vi "main.vi"() -> ()   [LabVIEW 2019]
uses:
  <vilib>/myRIO/Instrument Drivers/Onboard IO/I2C/typedefs/I2C Transfer Rate.ctl
  <vilib>/myRIO/Instrument Drivers/Onboard IO/I2C/I2C.lvlib
  <vilib>/myRIO/Instrument Drivers/Onboard IO/I2C/typedefs/I2C User Configuration.ctl
  <vilib>/myRIO/Instrument Drivers/Onboard IO/I2C/typedefs/I2C Configuration.ctl
  <vilib>/myRIO/Common/Instrument Driver Framework/myRIO v1.0/I2C/typedefs/I2C Channels Enum.ctl
  <vilib>/myRIO/Common/Instrument Driver Framework/Utilities/typedefs/Generic FPGA Reference.ctl
  <vilib>/myRIO/Common/Instrument Driver Framework/Utilities/typedefs/myRIO v1.0 Reference.ctl
  <vilib>/myRIO/Common/Instrument Driver Framework/Utilities/typedefs/Hardware Version Enum.ctl
  <vilib>/myRIO/Common/Instrument Driver Framework/Utilities/typedefs/myRIO Generic Hardware Reference.ctl
  <vilib>/myRIO/Instrument Drivers/Onboard IO/I2C/typedefs/I2C Reference.ctl
  <vilib>/myRIO/Instrument Drivers/Onboard IO/I2C/vis/Configure.vi
  <vilib>/userDefined/High Color/nirio_resource_hc.ctl
  <vilib>/myRIO/Common/Instrument Driver Framework/myRIO v1.0/I2C/vis/myRIO v1.1 Open I2C.vi
  <vilib>/myRIO/Instrument Drivers/Onboard IO/I2C/vis/myRIO I2C Open.xnode
  <vilib>/myRIO/Common/Instrument Driver Framework/Utilities/vis/Is FPGA Ref Available.vi
  <vilib>/myRIO/Express VI/Onboard IO/I2C/I2C Express VI.xnode
  <vilib>/Platform/TimedLoop/XDataNode/wakeup.ctl
  <vilib>/Platform/TimedLoop/XDataNode/XDNodeRunTimeDep.lvlib
  <vilib>/Platform/TimedLoop/XDataNode/nitl_modes.ctl
  <vilib>/Platform/TimedLoop/XDataNode/timing_clust.ctl
  <vilib>/platform/TimedLoop/XDataNode/XDataNode.xnode
  <vilib>/myRIO/Instrument Drivers/Onboard IO/I2C/vis/Write Read.vi
  <vilib>/myRIO/Instrument Drivers/Onboard IO/I2C/vis/Write.vi
  <vilib>/myRIO/Instrument Drivers/Utilities/Utilities.lvlib
  <vilib>/myRIO/Instrument Drivers/Onboard IO/PWM/PWM.lvlib
  <vilib>/myRIO/Instrument Drivers/Onboard IO/PWM/vis/myRIO PWM Open.xnode
  <vilib>/myRIO/Instrument Drivers/Onboard IO/PWM/typedefs/PWM Reference.ctl
  <vilib>/myRIO/Instrument Drivers/Onboard IO/PWM/typedefs/PWM Configuration.ctl
  <vilib>/myRIO/Common/Instrument Driver Framework/myRIO v1.0/PWM/typedefs/PWM Channels Enum.ctl
  <vilib>/myRIO/Common/Instrument Driver Framework/myRIO v1.0/PWM/vis/myRIO v1.1 Open PWM.vi
  OneDrive/Documents/LabVIEW Data/MathScriptVIs/MCStatic_41946317732_98df4686c37d1a1eae0c5985e9f7cbe2.vi
  <vilib>/imath/engines/lvmath2/RunTimeEngine/ArithmeticOperatorToken/NIMS_ArithmeticOperator_multmx.vi
  <vilib>/imathl/engines/lvmath/Functions/Error Handling/Create Error.vi
  <vilib>/imath/engines/lvmath/Functions/Error Handling/MergeErrorsWrapper.vi
  <vilib>/imath/engines/lvmath2/RunTimeEngine/CommandStatement/MC_CommandStatement_break.vi
  OneDrive/Documents/LabVIEW Data/MathScriptVIs/MCStatic_41946317732_460fc674ac509ba7029ac98c4ab25738.vi
  <vilib>/imath/engines/lvmath2/RunTimeEngine/ArithmeticOperatorToken/NIMS_ArithmeticOperator_minus.vi
  <vilib>/imath/engines/lvmath2/RunTimeEngine/ErrorHandling/NIMS_Create Error From Enums.vi
  <vilib>/imath/engines/lvmath2/RunTimeEngine/BuiltInFunctions/abs/NIMS_abs(signed).vi
  <vilib>/imath/engines/lvmath2/RunTimeEngine/BuiltInFunctions/max/1 input/NIMS_max(RM).vi
  <vilib>/imath/engines/lvmath2/RunTimeSupport/NIMS_Get Scalar_w Error.vi
  <vilib>/imath/engines/lvmath2/RunTimeEngine/BuiltInFunctions/eye/NIMS_M=eye(I32).vi
  <vilib>/imath/engines/lvmath2/RunTimeEngine/ArithmeticOperatorToken/NIMS_ArithmeticOperator_plus.vi
  <vilib>/imath/engines/lvmath2/RunTimeEngine/BuiltInFunctions/all/NIMS_all(GM).vi
  <vilib>/imath/engines/lvmath2/RunTimeEngine/ArithmeticOperatorToken/NIMS_ArithmeticOperator_powermx(M,M).vi
  <vilib>/imath/engines/lvmath2/RunTimeEngine/CommandStatement/NIMS_CommandStatement_MaskErr.vi
  <vilib>/imath/engines/lvmath2/RunTimeEngine/ErrorHandling/NIMS_Finalize Error.vi
  Analytic_Jacobian_Mag_cir_array_test.m
  PM_forward_field.m
  <vilib>/Utility/file.llb/Write Delimited Spreadsheet (DBL).vi
  <vilib>/imath/engines/lvmath2/RunTimeEngine/BuiltInFunctions/max/1 input/NIMS_max(CM).vi
  <vilib>/imath/engines/lvmath2/RunTimeEngine/BuiltInFunctions/diag/NIMS_diag.vi
  <vilib>/imath/engines/lvmath2/RunTimeEngine/BuiltInFunctions/is_finite/NIMS_is_finite.vi
  <vilib>/imath/engines/lvmath2/RunTimeEngine/BuiltInFunctions/length/NIMS_length(GV).vi
  <vilib>/imath/engines/lvmath2/RunTimeEngine/BuiltInFunctions/norm/NIMS_norm(GM,DBL).vi
  <vilib>/imath/engines/lvmath2/RunTimeEngine/ArithmeticOperatorToken/NIMS_ArithmeticOperator_rightdivmx(C,C).vi
  <vilib>/imath/engines/lvmath2/RunTimeEngine/BuiltInFunctions/max/2 inputs/NIMS_max(CG,CG)-no size check.vi
  <vilib>/imath/engines/lvmath2/RunTimeEngine/NodeEndStatement/NIMS_NodeEndStatement_Output.vi
  <vilib>/imath/engines/lvmath2/RunTimeEngine/ArithmeticOperatorToken/NIMS_ArithmeticOperator_rightdiv.vi
  <vilib>/imath/engines/lvmath2/RunTimeEngine/ArithmeticOperatorToken/NIMS_ArithmeticOperator_leftdivmx(C,C).vi
  <vilib>/imath/engines/lvmath2/RunTimeEngine/BuiltInFunctions/mirrorh/NIMS_mirrorh(GM).vi
  <vilib>/imath/engines/lvmath2/RunTimeEngine/RowToken/NIMS_RowToken_M_M.vi
  <vilib>/Utility/file.llb/Write Delimited Spreadsheet (string).vi
  <vilib>/myRIO/Express VI/Onboard IO/PWM/PWM Express VI.xnode
  <vilib>/myRIO/Instrument Drivers/Onboard IO/PWM/vis/Set Duty Cycle and Frequency.vi
panel:
  out "pm_hat_opt 2":dbl[][](array[numeric])
  in  "stop 2":bool
  out "Combined Output":cluster{dbl, dbl, dbl, dbl, dbl, dbl}(graph) caption="Waveform Chart"
  out "MUX 2":cluster{dbl, dbl, dbl}(graph) caption="Waveform Chart"
  out "MUX 1":cluster{dbl, dbl, dbl}(graph) caption="Waveform Chart"
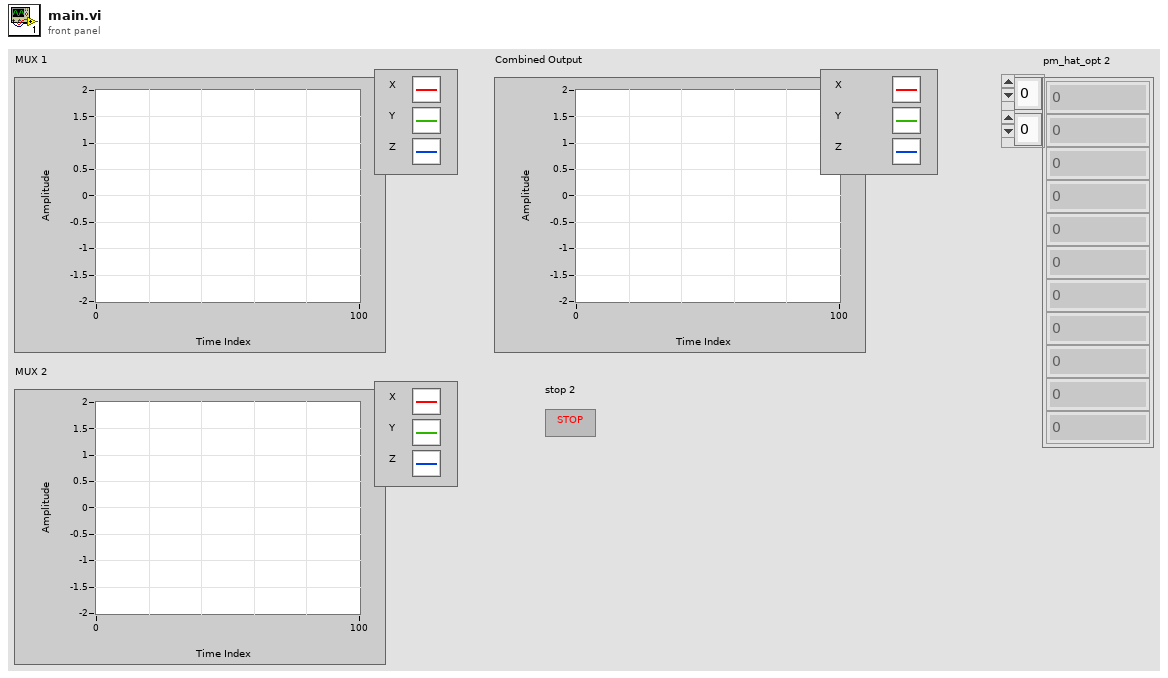
[diagram p1: front panel]
types:
  T1 = typedef "I2C.lvlib/I2C Reference.ctl" = cluster{"myRIO Reference":T2, "I2C Channels Enum":T6, "I2C Configuration":T7}
  T2 = typedef "myRIO Generic Hardware Reference.ctl" = cluster{"myRIO Model":T3, "myRIO Hardware Reference":T4}
  T3 = typedef "Hardware Version Enum.ctl" = enum16{"Unknown", "myRIO-1900", "myRIO-1950", "roboRIO", "NI ELVIS RIO CM", "ELVIS III"}
  T4 = typedef "myRIO v1.0 Reference.ctl" = cluster{"Generic FPGA Reference":T5, "Allow multiple opens":bool}
  T5 = typedef "Generic FPGA Reference.ctl" = refnum<k20>
  T6 = typedef "I2C Channels Enum.ctl" = enum16{"Not Connected", "A/I2C", "B/I2C", "I2C/I2C"}
  T7 = typedef "I2C.lvlib/I2C Configuration.ctl" = cluster{"I2C Transfer Rate":T8}
  T8 = typedef "I2C.lvlib/I2C Transfer Rate.ctl" = enum16{"Standard mode (100 kbps)", "Fast mode (400 kbps)"}
  T9 = typedef "I2C.lvlib/I2C User Configuration.ctl" = cluster{"I2C Transfer Rate":T8}
  T10 = typedef "nirio_resource_hc.ctl" = tag
  T11 = typedef "PWM.lvlib/PWM Reference.ctl" = cluster{"myRIO Reference":T2, "PWM Channels Enum":T12, "PWM Configuration":T13}
  T12 = typedef "PWM Channels Enum.ctl" = enum16{"Not Connected", "C/PWM0", "C/PWM1", "A/PWM0", "A/PWM1", "A/PWM2", "A/PWM3", "A/PWM4", "A/PWM5", "A/PWM6", "A/PWM7", "A/PWM8", "A/PWM9", "A/PWM10", "A/PWM11", "A/PWM12", "A/PWM13", "A/PWM14", "A/PWM15", "A/PWM16", "A/PWM17", "A/PWM18", "A/PWM19", "B/PWM0", "B/PWM1", "B/PWM2", "B/PWM3", "B/PWM4", "B/PWM5", "B/PWM6", "B/PWM7", "B/PWM8", "B/PWM9", "B/PWM10", "B/PWM11", "B/PWM12", "B/PWM13", "B/PWM14", "B/PWM15", "B/PWM16", "B/PWM17", "B/PWM18", "B/PWM19", "PWM/PWM0", "PWM/PWM1", "PWM/PWM2", "PWM/PWM3", "PWM/PWM4", "PWM/PWM5", "PWM/PWM6", "PWM/PWM7", "PWM/PWM8", "PWM/PWM9"}
  T13 = typedef "PWM.lvlib/PWM Configuration.ctl" = cluster{"Frequency":dbl, "Duty Cycle":dbl}
  T14 = typedef "XDNodeRunTimeDep.lvlib/timing_clust.ctl" = cluster{"Expected End [f-1]":u64, "Actual End [f-1]":u64, "Finished Late? [f-1]":bool, "Expected End [i-1]":u64, "Actual End [i-1]":u64, "Finished Late? [i-1]":bool, "Expected Start [i]":u64, "Actual Start [i]":u64, "Expected Start [f]":u64, "Actual Start [f]":u64, "Source Name":string, "Structure Name":string, "Period":i64, "Deadline":i64, "Offset":i64, "Start":i64, "Priority":i32, "Timeout":i32, "Mode":T15, "Wakeup Reason":T16, "Error":errorcluster, "Source Type":string, "Secondary Source Type":string, "Global End Time":u64, "Global Start Time":u64, "Frame Duration":u64, "Iteration Duration":u64, "Assigned CPU":i32, "I/O Scan Engine Mode":u32}
  T15 = typedef "XDNodeRunTimeDep.lvlib/nitl_modes.ctl" = enum32{"No Change", "Process missed periods, maintain original phase", "Discard missed periods, maintain original phase", "Process missed periods, ignore original phase", "Discard missed periods, ignore original phase"}
  T16 = typedef "XDNodeRunTimeDep.lvlib/wakeup.ctl" = enum32{"Normal", "Aborted", "Asynchronous wakeup", "Timing source error", "Timed loop error", "Timeout"}
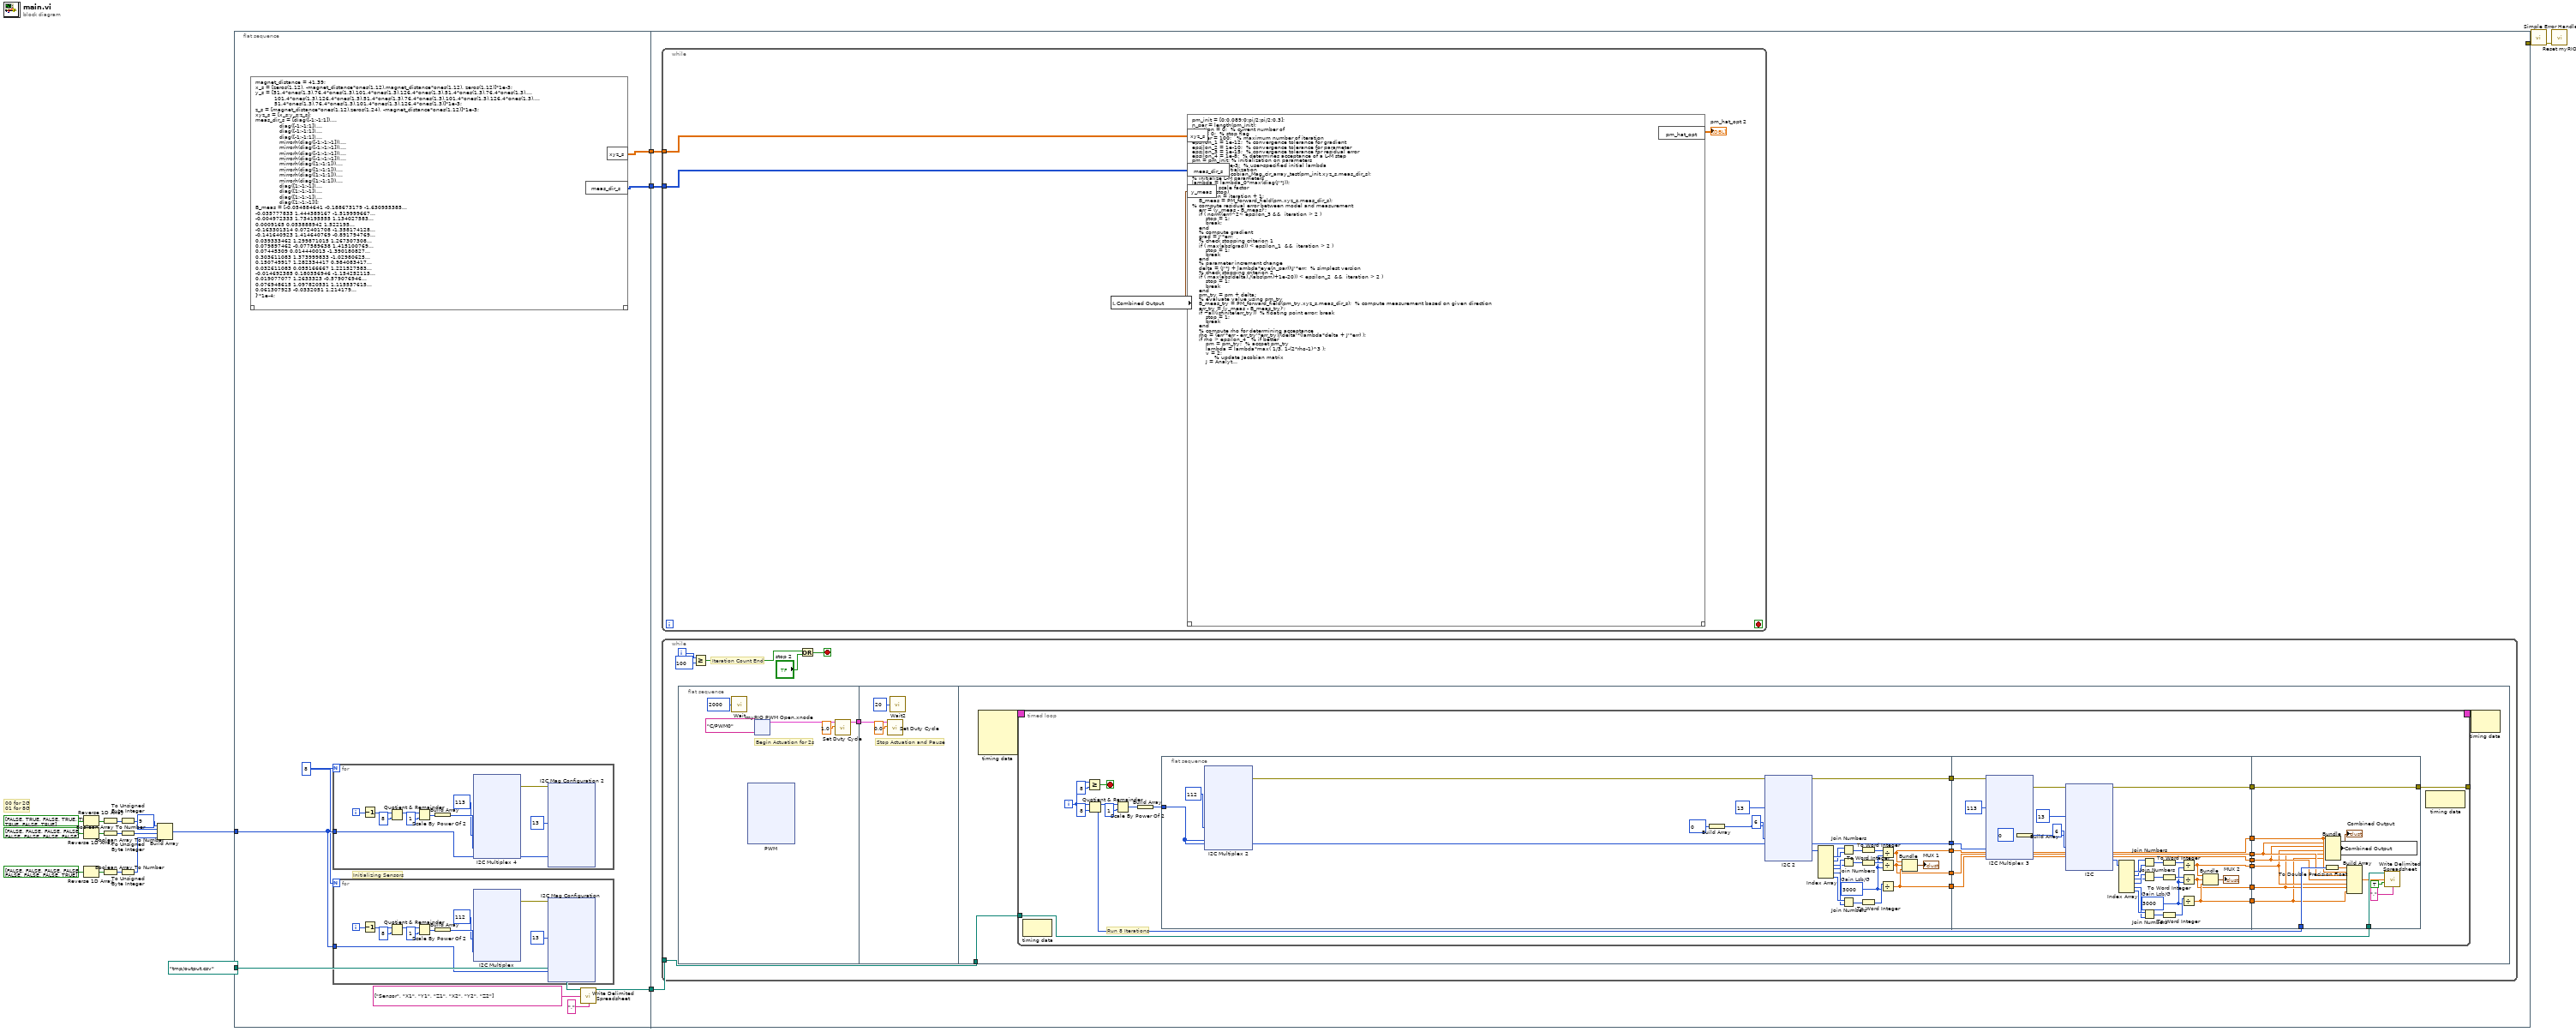
[diagram p0: block diagram]
diagram:
  # "00 for 2G\n01 for 8G"
  n1 = Reverse 1D Array(array=bool[] [FALSE, TRUE, FALSE, TRUE, TRUE, TRUE, FALSE, TRUE]) -> (reversed array=w19:bool[])
  n2 = Reverse 1D Array(array=bool[] [FALSE, FALSE, FALSE, FALSE, FALSE, FALSE, FALSE, FALSE]) -> (reversed array=w18:bool[])
  n3 = Reverse 1D Array(array=bool[] [FALSE, FALSE, FALSE, FALSE, FALSE, FALSE, FALSE, TRUE]) -> (reversed array=w16:bool[])
  n4 = Boolean Array To Number(Boolean array=w19) -> (number=w13:u32)
  n5 = Boolean Array To Number(Boolean array=w18) -> (number=w12:u32)
  n6 = Boolean Array To Number(Boolean array=w16) -> (number=w11:u32)
  n7 = To Unsigned Byte Integer(number=w13) -> (unsigned 8bit integer=w10:u8)
  n8 = To Unsigned Byte Integer(number=w12) -> (unsigned 8bit integer=w9:u8)
  n9 = To Unsigned Byte Integer(number=w11) -> (unsigned 8bit integer=w8:u8)
  n10 = Build Array(u8 9 ("address"), w10, w9, w8) -> (w7:u8[])
  n11 = flat-sequence {
    tunnel: [w28] -> w3
    tunnel: path "/tmp/output.csv" ("file path (dialog if empty)") -> [w24]
    tunnel: w7 -> [w27]
    tunnel: [w22] -> w2
    tunnel: [w21] -> w1
    tunnel: [_] -> w6
    tunnel: w3 -> [w457]
    tunnel: w2 -> [w456]
    tunnel: w1 -> [w455]
    frame #0 {
      w26 = 8
      # "Initializing Sensors"
      n12 = mathscript code="magnet_distance = 41.39;\nx_s = [zeros(1,12), -magnet_distance*ones(1,12),magnet_distance*ones(1,12), zeros(1,12)]*1e-3; \ny_s = [51.4*ones(1,3),76.4*ones(1,3),101.4*ones(1,3),126.4*ones(1,3),51.4*ones(1,3),76.4*ones(1,3),...\n           101.4*ones(1,3),126.4*ones(1,3),51.4*ones(1,3),76.4*ones(1,3),101.4*ones(1,3),126.4*ones(1,3),...\n           51.4*ones(1,3),76.4*ones(1,3),101.4*ones(1,3),126.4*ones(1,3)]*1e-3; \nz_s = [magnet_distance*ones(1,12),zeros(1,24), -magnet_distance*ones(1,12)]*1e-3; \nxyz_s = [x_s;y_s;z_s];  \nmeas_dir_s = [diag([-1;-1;1]),...\n              diag([-1;-1;1]),...\n              diag([-1;-1;1]),...\n              diag([-1;-1;1]),...\n              mirrorh(diag([-1;-1;-1])),...\n              mirrorh(diag([-1;-1;-1])),...\n              mirrorh(diag([-1;-1;-1])),...\n              mirrorh(diag([-1;-1;-1])),...\n              mirrorh(diag([1;-1;1])),...\n              mirrorh(diag([1;-1;1])),...\n              mirrorh(diag([1;-1;1])),...\n              mirrorh(diag([1;-1;1])),...\n              diag([1;-1;-1]),...\n              diag([1;-1;-1]),...\n              diag([1;-1;-1]),...\n              diag([1;-1;-1])];\nB_meas = [-0.054884641\t-0.188673179\t-1.630955385...\n-0.035777833\t1.444389167\t-1.519999667...\n-0.004972333\t1.734195555\t1.134027583...\n0.0009165\t0.053888942\t1.522195...\n-0.163301314\t0.072401708\t-1.358174128...\n-0.141640923\t1.414640769\t-0.891794769...\n0.039333462\t1.299871015\t1.267307308...\n0.079897462\t-0.077589638\t1.415100769...\n0.07445309\t0.014440013\t-1.390180827...\n0.303611083\t1.373999833\t-1.02980625...\n0.150749917\t1.282334417\t0.984083417...\n0.032611083\t0.055166667\t1.221527583...\n-0.014692385\t0.180356946\t-1.154252115...\n0.019077077\t1.2633323\t-0.579076946...\n0.076948615\t1.097820531\t1.115537615...\n0.061307923\t-0.0332051\t1.214179...\n]'*1e-4;"() -> ("meas_dir_s"=w22:i32[][], "xyz_s"=w21:dbl[][])  [unwired: 1 in, 1 out]
      n13 = for {
        N: w26 -> [_]
        tunnel: w27 -> [w288]
        i -> [w282]
        n14 = Decrement(x=w282) -> (x-1=w281:i32)
        n15 = Quotient & Remainder(x=w281, y=8) -> (x-y*floor(x/y)=w283:i32)  [unwired: 1 out]
        n16 = Scale By Power Of 2(n=w283, x=1) -> (x*2^n=w285:i32)
        n17 = Build Array(w285) -> (w291:i32[])
        n18 = xnode "I2C Multiplex 4"("Slave Address (7-bit)"=u8 113, "Bytes to Write"=w291) -> ("error out"=w290:errorcluster)  [unwired: 1 in]
        n19 = xnode "I2C Mag Configuration 2"("Slave Address (7-bit)"=u8 13, "Bytes to Write"=w288, "error in (no error)"=w290) -> ()  [unwired: 1 out]
      }
      n20 = for {
        N: w26 -> [_]
        tunnel: w27 -> [w375]
        i -> [w369]
        n21 = Decrement(x=w369) -> (x-1=w368:i32)
        n22 = Quotient & Remainder(x=w368, y=8) -> (x-y*floor(x/y)=w370:i32)  [unwired: 1 out]
        n23 = Scale By Power Of 2(n=w370, x=1) -> (x*2^n=w372:i32)
        n24 = Build Array(w372) -> (w378:i32[])
        n25 = xnode "I2C Multiplex"("Slave Address (7-bit)"=u8 112, "Bytes to Write"=w378) -> ("error out"=w377:errorcluster)  [unwired: 1 in]
        n26 = xnode "I2C Mag Configuration"("Slave Address (7-bit)"=u8 13, "Bytes to Write"=w375, "error in (no error)"=w377) -> ()  [unwired: 1 out]
      }
      n27 = call-poly <vilib>:"Write Delimited Spreadsheet.vi"("file path (dialog if empty)"=w24, "1D data"=string[] ["Sensor", "X1", "Y1", "Z1", "X2", "Y2", "Z2"], "delimiter (\\t)"="," ("delimiter (\\t)")) -> ("new file path (Not A Path if cancelled)"=w28:path)  [unwired: 11 in, 1 out]
    }
    frame #1 {
      n28 = while {
        tunnel: w456 -> [w459]
        tunnel: w455 -> [w458]
        stop <- _ stop-if-true
        n29 = local read "Combined Output"() -> (w461:cluster{dbl, dbl, dbl, dbl, dbl, dbl})
        n30 = mathscript code="pm_init = [0;0.089;0;pi/2;pi/2;0.3];\nn_par = length(pm_init);\niteration = 0;  % current number of \nstop = 0;  % stop flag\nMaxIter = 100;   % maximum number of iteration\nepsilon_1 = 1e-12;  % convergence tolerance for gradient\nepsilon_2 = 1e-10;  % convergence tolerance for parameter\nepsilon_3 = 1e-15;  % convergence tolerance for residual error\nepsilon_4 = 1e-8;  % determines acceptance of a L-M step\npm = pm_init; % initialization on parameters\nlambda_0 = 1e-3;  % user-specified initial lambda\n% Jacobian initialization\nJ = Analytic_Jacobian_Mag_cir_array_test(pm_init,xyz_s,meas_dir_s);\n% initialize L-M parameters\nlambda = lambda_0*max(diag(J'*J));\nv = 2;  % scale factor\nwhile ( ~stop)\n    iteration = iteration + 1;\n    B_meas = PM_forward_field(pm,xyz_s,meas_dir_s);\n% compute residual error between model and measurement\n    err = (y_meas - B_meas)';\n    if ( norm(err)^2< epsilon_3 &&  iteration > 2 )\n        stop = 1;\n        break;\n    end\n    % compute gradient\n    grad = J'*err;\n    % check stopping criterion 1\n    if ( max(abs(grad)) < epsilon_1  &&  iteration > 2 )\n        stop = 1;\n        break\n    end\n    % parameter increment change\n    delta = (J'*J + lambda*eye(n_par))\\J'*err;  % simplest version\n    % check stopping criterion 2 \n    if ( max(abs(delta)./(abs(pm)+1e-20)) < epsilon_2  &&  iteration > 2 )\n        stop = 1;\n        break\n    end\n    pm_try = pm + delta;\n    % evaluate value using pm_try\n    B_meas_try = PM_forward_field(pm_try,xyz_s,meas_dir_s);  % compute measurement based on given direction\n    err_try = (y_meas - B_meas_try)';\n    if ~all(isfinite(err_try))  % floating point error; break\n        stop = 1;\n        break\n    end\n    % compute rho for determining acceptance\n    rho = (err'*err - err_try'*err_try)/(delta'*(lambda*delta + J'*err) );\n    if rho > epsilon_4   % if better\n        pm = pm_try;  % accpet pm_try\n        lambda = lambda*max( 1/3, 1-(2*rho-1)^3 );\n        v = 2;\n             % update Jacobian matrix\n        J = Analytic_Jacobian_Mag_cir_array_test(pm,xyz_s,meas_dir_s);\n    else      % if not better\n        lambda = lambda*v;\n        v = 2*v;\n    end\n    if ( iteration == MaxIter )\n        stop = 1;\n    end\nend\n\npm_hat_opt = pm;"("meas_dir_s"=w459, "xyz_s"=w458, "y_meas"=w461) -> ("pm_hat_opt"=→"pm_hat_opt 2":dbl[][])  [unwired: 1 in, 1 out]
      }
      n31 = while {
        tunnel: w457 -> [w1508]
        i -> [w1507]
        stop <- w1503 stop-if-true
        # "Iteration Count End"
        n32 = flat-sequence {
          tunnel: [w1510] -> w1509
          tunnel: w1509 -> [w1567]
          tunnel: w1508 -> [w1569]
          frame #0 {
            # "Begin Actuation for 2s"
            n33 = call "Wait"("Count(mSec)"=u32 2000) -> ()  [unwired: 1 out]
            n34 = xnode "PWM"() -> ()  [unwired: 3 in, 1 out]
            n35 = xnode "myRIO PWM Open.xnode"("Channel Name"=tag "C/PWM0") -> ("PWM Ref Out"=w1514:T11)  [unwired: 2 in, 1 out]
            n36 = call <vilib>:"Set Duty Cycle.vi"("Duty Cycle"=1.0, "PWM Ref In"=w1514) -> ("PWM Ref Out"=w1510:T11)  [unwired: 7 in, 1 out]
          }
          frame #1 {
            # "Stop Actuation and Pause"
            n37 = call <vilib>:"Set Duty Cycle.vi"("Duty Cycle"=0.0, "PWM Ref In"=w1567) -> ()  [unwired: 7 in, 2 out]
            n38 = call "Wait2"("Count(mSec)"=u32 20) -> ()  [unwired: 1 out]
          }
          frame #2 {
            n39 = node-c288() -> (w1571:T14)  [unwired: 4 in]
            n40 = timed-loop {
              timing: w1571 -> [_]
              timing-out: [_] -> w1570
              tunnel: [w1589] -> _
              tunnel: w1569 -> [w1576]
              i -> [w1573]
              stop <- w1572 stop-if-true
              # "Run 8 Iterations"
              n41 = node-c288() -> ()  [unwired: 1 in, 1 out]
              n42 = Greater Or Equal?(x=w1573, y=8) -> (x >= y?=w1572:bool)
              n43 = Quotient & Remainder(x=w1573, y=8) -> (x-y*floor(x/y)=w1575:i32)  [unwired: 1 out]
              n44 = Scale By Power Of 2(n=w1575, x=1) -> (x*2^n=w1577:i32)
              n45 = Build Array(w1577) -> (w1592:i32[])
              n46 = flat-sequence {
                tunnel: w1592 -> [w1600]
                tunnel: [w1600] -> w1590
                tunnel: [w1598] -> w1588
                tunnel: [w1597] -> w1582
                tunnel: [w1596] -> w1580
                tunnel: [w1595] -> w1578
                tunnel: w1590 -> [w1708]
                tunnel: w1588 -> [w1705]
                tunnel: [w1706] -> w1587
                tunnel: [w1704] -> w1586
                tunnel: [w1703] -> w1585
                tunnel: [w1702] -> w1584
                tunnel: [w1701] -> w1583
                tunnel: w1582 -> [w1701]
                tunnel: [w1700] -> w1581
                tunnel: w1580 -> [w1700]
                tunnel: [w1699] -> w1579
                tunnel: w1578 -> [w1699]
                tunnel: [w1819] -> w1589
                tunnel: w1587 -> [w1819]
                tunnel: w1586 -> [w1810]
                tunnel: w1585 -> [w1808]
                tunnel: w1584 -> [w1809]
                tunnel: w1583 -> [w1811]
                tunnel: w1581 -> [w1813]
                tunnel: w1579 -> [w1814]
                tunnel: w1575 -> [w1818]
                tunnel: w1576 -> [w1816]
                frame #0 {
                  w1609 = i16 3000  # Gain Lsb/G
                  n47 = xnode "I2C Multiplex 2"("Slave Address (7-bit)"=u8 112, "Bytes to Write"=w1600) -> ("error out"=w1599:errorcluster)  [unwired: 1 in]
                  n48 = Build Array(u8 0) -> (w1613:u8[])
                  n49 = xnode "I2C 2"("Slave Address (7-bit)"=u8 13, "Bytes to Write"=w1613, "Byte Count"=u32 6, "error in (no error)"=w1599) -> ("Bytes Read"=w1616:u8[], "error out"=w1598:errorcluster)
                  n50 = Index Array(array=w1616) -> (element #1=w1608:u8, element #2=w1607:u8, element #3=w1605:u8, element #4=w1606:u8, element #5=w1603:u8, element #6=w1604:u8)  [unwired: 6 in]
                  n51 = Join Numbers(hi=w1607, lo=w1608) -> ((hi.lo)=w1619:u16)
                  n52 = Join Numbers(hi=w1606, lo=w1605) -> ((hi.lo)=w1617:u16)
                  n53 = Join Numbers(hi=w1604, lo=w1603) -> ((hi.lo)=w1618:u16)
                  n54 = To Word Integer(number=w1619) -> (16bit integer=w1612:i16)
                  n55 = To Word Integer(number=w1617) -> (16bit integer=w1611:i16)
                  n56 = To Word Integer(number=w1618) -> (16bit integer=w1610:i16)
                  n57 = Divide(x=w1612, y=w1609) -> (x/y=w1595:dbl)
                  n58 = Divide(x=w1611, y=w1609) -> (x/y=w1596:dbl)
                  n59 = Divide(x=w1610, y=w1609) -> (x/y=w1597:dbl)
                  n60 = Bundle(w1595, w1596, w1597) -> (→"MUX 1":cluster{dbl, dbl, dbl})  [unwired: 1 in]
                }
                frame #1 {
                  w1717 = i16 3000  # Gain Lsb/G
                  n61 = xnode "I2C Multiplex 3"("Slave Address (7-bit)"=u8 113, "Bytes to Write"=w1708, "error in (no error)"=w1705) -> ("error out"=w1707:errorcluster)
                  n62 = Build Array(u8 0) -> (w1721:u8[])
                  n63 = xnode "I2C"("Slave Address (7-bit)"=u8 13, "Bytes to Write"=w1721, "Byte Count"=u32 6, "error in (no error)"=w1707) -> ("Bytes Read"=w1724:u8[], "error out"=w1706:errorcluster)
                  n64 = Index Array(array=w1724) -> (element #1=w1716:u8, element #2=w1715:u8, element #3=w1713:u8, element #4=w1714:u8, element #5=w1711:u8, element #6=w1712:u8)  [unwired: 6 in]
                  n65 = Join Numbers(hi=w1715, lo=w1716) -> ((hi.lo)=w1727:u16)
                  n66 = Join Numbers(hi=w1714, lo=w1713) -> ((hi.lo)=w1725:u16)
                  n67 = Join Numbers(hi=w1712, lo=w1711) -> ((hi.lo)=w1726:u16)
                  n68 = To Word Integer(number=w1727) -> (16bit integer=w1720:i16)
                  n69 = To Word Integer(number=w1725) -> (16bit integer=w1719:i16)
                  n70 = To Word Integer(number=w1726) -> (16bit integer=w1718:i16)
                  n71 = Divide(x=w1720, y=w1717) -> (x/y=w1704:dbl)
                  n72 = Divide(x=w1719, y=w1717) -> (x/y=w1702:dbl)
                  n73 = Divide(x=w1718, y=w1717) -> (x/y=w1703:dbl)
                  n74 = Bundle(w1704, w1702, w1703) -> (→"MUX 2":cluster{dbl, dbl, dbl})  [unwired: 1 in]
                }
                frame #2 {
                  n75 = To Double Precision Float(number=w1818) -> (double precision float=w1815:dbl)
                  n76 = Bundle(w1814, w1813, w1811, w1810, w1809, w1808) -> (w1806:cluster{dbl, dbl, dbl, dbl, dbl, dbl})  [unwired: 1 in]
                  "Combined Output" <- w1806
                  n77 = local write "Combined Output"(w1806) -> ()
                  n78 = Build Array(w1815, w1814, w1813, w1811, w1810, w1809, w1808) -> (w1807:dbl[])
                  n79 = call-poly <vilib>:"Write Delimited Spreadsheet.vi"("file path (dialog if empty)"=w1816, "1D data"=w1807, "append to file? (new file:F)"=TRUE, "delimiter (\\t)"="," ("delimiter (\\t)")) -> ()  [unwired: 10 in, 2 out]
                }
              }
              n80 = node-c288() -> ()  [unwired: 1 in, 1 out]
            }
            n81 = node-c288(w1570) -> ()  [unwired: 1 out]
          }
        }
        n82 = Greater Or Equal?(x=w1507, y=100) -> (x >= y?=w1505:bool)
        n83 = Or(x=w1505, y="stop 2") -> (x .or. y?=w1503:bool)
      }
    }
  }
  n84 = call <vilib>:"Simple Error Handler.vi"("error in (no error)"=w6) -> ("error out"=w5:errorcluster)  [unwired: 4 in, 4 out]
  n85 = call <vilib>:"Reset myRIO.vi"("error in (no error)"=w5) -> ()  [unwired: 10 in, 1 out]
